vi "save_tracks_to_mat.vi"(3 "Max Spatial Drift Since Experiment Start (mm)":dbl, 5 "Max Spatial Drift Since Last Calibration (mm)":dbl, 7 "DecodedCameraFrames":i32[](array[numeric]), 8 "error in":errorcluster, 11 "Completed Tracks":T1[](array[typedef])) -> (0 "error out":errorcluster, 1 "Last Buffer":i32, 2 "total time elapsed (ms)":i32)   [LabVIEW 2019]
uses:
  WormTrackCluster.ctl
  StimulusObject.lvclass
  TrackTerminationReasonEnum.ctl
  WormTrackSavingCluster.ctl
  TimestampsFunctionalGlobalOperations.ctl
  <vilib>/addons/h5labview2/file/H5Fmode.ctl
  StimulusObject.lvclass/StimulusObject.ctl
  ParametersGlobal.vi
  <vilib>/addons/h5labview2/file/H5F.lvlib
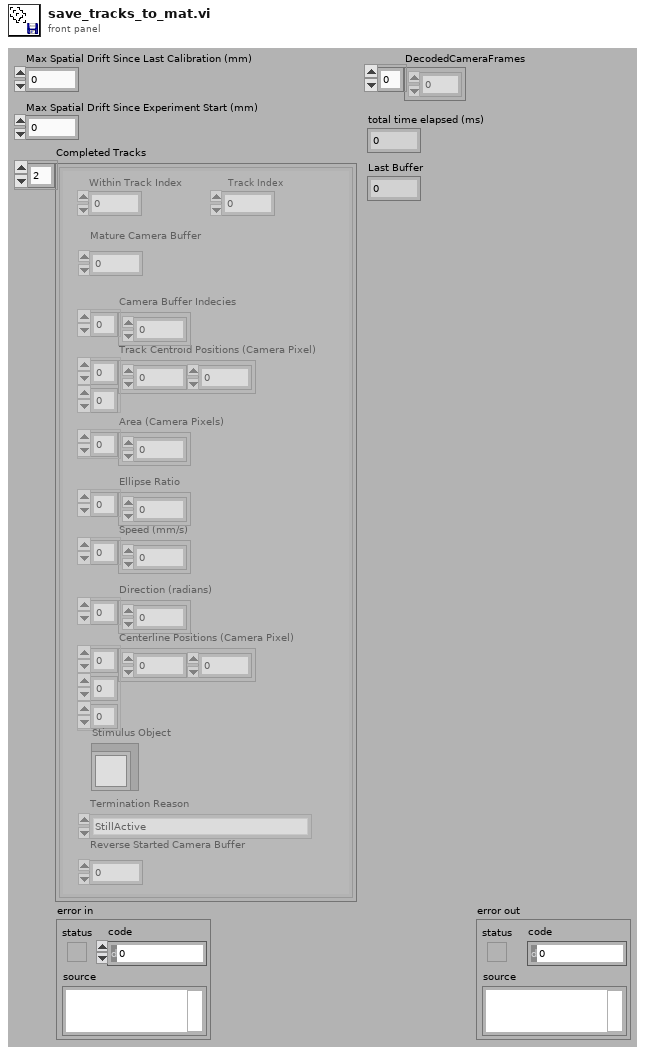
[diagram p1: front panel]
types:
  T1 = typedef "WormTrackCluster.ctl" = cluster{"Track Centroid Positions (Camera Pixel)":sgl[][], "Within Track Index":i32, "Camera Buffer Indecies":i32[], "Area (Camera Pixels)":i32[], "Speed (mm/s)":sgl[], "Direction (radians)":sgl[], "Centerline Positions (Camera Pixel)":sgl[][][], "Ellipse Ratio":sgl[], "Stimulus Object":refnum<class "StimulusObject.lvclass">, "Termination Reason":T2, "Track Index":i32, "Mature Camera Buffer":i32, "Reverse Started Camera Buffer":i32}
  T2 = typedef "TrackTerminationReasonEnum.ctl" = enum16{"StillActive", "MaxDisplacement", "NoBlobsLeft", "AreaIncrease", "AreaDecrease", "ExperimentEnded"}
  T3 = typedef "H5F.lvlib/H5Fmode.ctl" = enum16{"read-only", "read-write", "overwrite", "create new", "open or create"}
  T4 = typedef "TimestampsFunctionalGlobalOperations.ctl" = enum16{"Initialize", "Dump", "UpdateTime", "ReadTime"}
  T5 = typedef "WormTrackSavingCluster.ctl" = cluster{"Path":sgl[][], "Frames":i32[], "Size":i32[], "Speed":sgl[], "Direction":sgl[], "LabviewCenterline":sgl[][][], "EllipseRatio":sgl[], "TerminationReason":string, "WormIndex":i32, "MatureCameraBuffer":i32, "Stimulus":sgl[][]}
  T6 = typedef "IMAQ Image.ctl" = refnum<image>
  T7 = typedef "hid_t.ctl" = i32
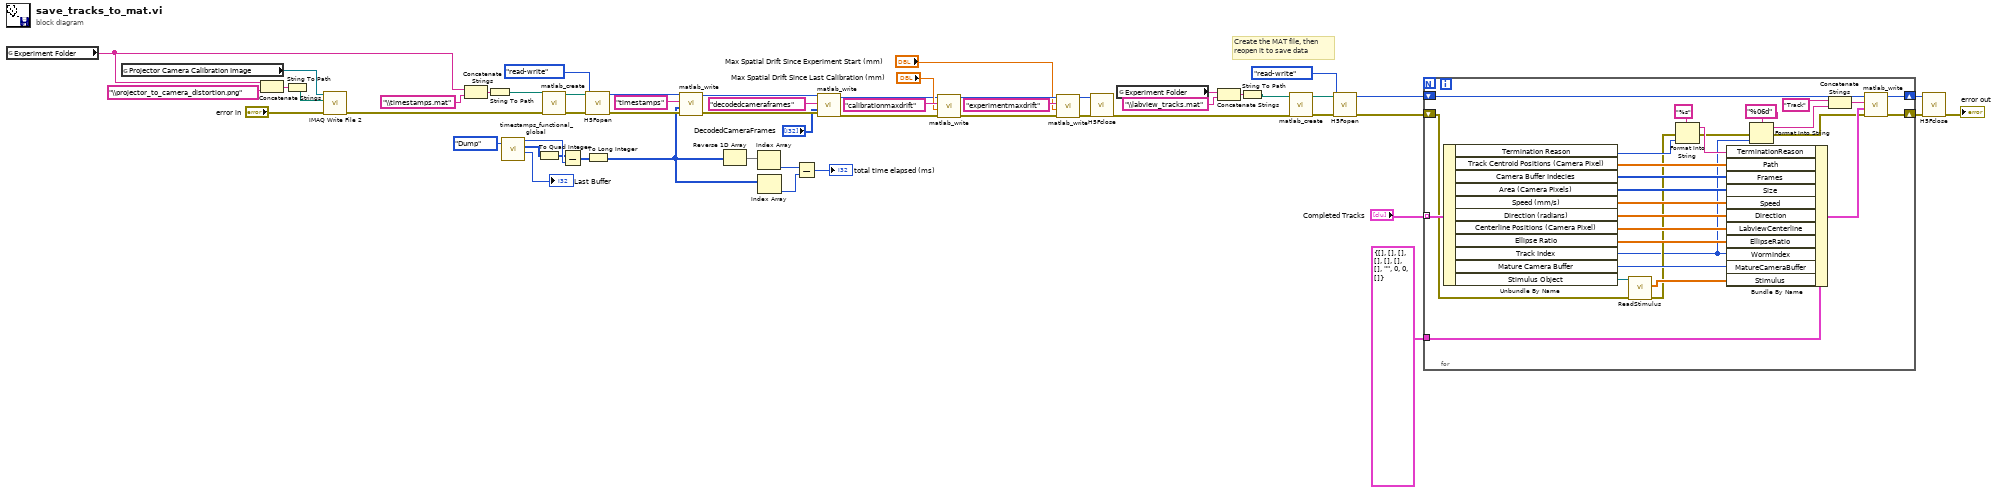
[diagram p0: block diagram]
diagram:
  # "Create the MAT file, then\nreopen it to save data"
  n1 = global read "ParametersGlobal.vi" "Experiment Folder"() -> (w11:string)
  n2 = global read "ParametersGlobal.vi" "Projector Camera Calibration Image"() -> (w13:T6)
  n3 = Concatenate Strings(w11, "\\projector_to_camera_distortion.png" ("string")) -> (w17:string)
  n4 = String To Path(string=w17) -> (path=w12:path)
  n5 = call-poly "IMAQ Write File 2"("error in (no error)"="error in", "File Path"=w12, "Image"=w13) -> ("error out"=w14:errorcluster)  [unwired: 7 in, 1 out]
  n6 = Concatenate Strings(w11, "\\timestamps.mat" ("string")) -> (w37:string)
  n7 = String To Path(string=w37) -> (path=w33:path)
  n8 = call "timestamps_functional_global.vi"("Operation"=TimestampsFunctionalGlobalOperations."Dump") -> ("Last Buffer"=→"Last Buffer":i32, "Timestamps"=w40:u32[], "Timestamp Out"=w41:u32)  [unwired: 4 in]
  n9 = To Quad Integer(1:w40) -> (0:w39:i64[])
  n10 = call "matlab_create.vi"("error in"=w14, "path in"=w33) -> ("error out"=w35:errorcluster, "path out"=w36:path)  [unwired: 4 in]
  n11 = Subtract(x=w39, y=w41) -> (x-y=w32:i64[])
  n12 = call <vilib>:"H5Fopen.vi"("error in (no error)"=w35, "mode (read-only)"=H5Fmode."read-write", "path"=w36) -> ("error out"=w29:errorcluster, "ref out"=w30:T7)  [unwired: 7 in]
  n13 = To Long Integer(number=w32) -> (32bit integer=w22:i32[])
  n14 = call "matlab_write.vi"("error in"=w29, "data in"=w22, "name"="timestamps", "ref in"=w30) -> ("error out"=w26:errorcluster, "ref out"=w25:T7)  [unwired: 2 in]
  n15 = Reverse 1D Array(array=w22) -> (reversed array=w23:i32[])
  n16 = Index Array(array=w23) -> (element=w21:i32)  [unwired: 1 in]
  n17 = Index Array(array=w22) -> (element=w20:i32)  [unwired: 1 in]
  n18 = Subtract(x=w21, y=w20) -> (x-y=→"total time elapsed (ms)":i32)
  n19 = call "matlab_write.vi"("error in"=w26, "data in"="DecodedCameraFrames", "name"="decodedcameraframes", "ref in"=w25) -> ("error out"=w8:errorcluster, "ref out"=w2:T7)  [unwired: 2 in]
  n20 = call "matlab_write.vi"("error in"=w8, "data in"="Max Spatial Drift Since Last Calibration (mm)", "name"="calibrationmaxdrift", "ref in"=w2) -> ("error out"=w6:errorcluster, "ref out"=w3:T7)  [unwired: 2 in]
  n21 = call "matlab_write.vi"("error in"=w6, "data in"="Max Spatial Drift Since Experiment Start (mm)", "name"="experimentmaxdrift", "ref in"=w3) -> ("error out"=w5:errorcluster, "ref out"=w4:T7)  [unwired: 2 in]
  n22 = call <vilib>:"H5Fclose.vi"("error in (no error)"=w5, "ref"=w4) -> ("error out"=w31:errorcluster)  [unwired: 9 in]
  n23 = global read "ParametersGlobal.vi" "Experiment Folder"() -> (w48:string)
  n24 = Concatenate Strings(w48, "\\labview_tracks.mat" ("string")) -> (w46:string)
  n25 = String To Path(string=w46) -> (path=w45:path)
  n26 = call "matlab_create.vi"("error in"=w31, "path in"=w45) -> ("error out"=w55:errorcluster, "path out"=w56:path)  [unwired: 4 in]
  n27 = call <vilib>:"H5Fopen.vi"("error in (no error)"=w55, "mode (read-only)"=H5Fmode."read-write", "path"=w56) -> ("error out"=w51:errorcluster, "ref out"=w52:T7)  [unwired: 7 in]
  n28 = for {
    shift-right: [w82] -> w49
    shift-left: w52 -> [w84]
    shift-right: [w83] -> w50
    shift-left: w51 -> [w63]
    tunnel: "Completed Tracks" -> [w79] mode=indexing
    tunnel: T5 {"Path"=[], "Frames"=[], "Size"=[], "Speed"=[], "Direction"=[], "LabviewCenterline"=[], "EllipseRatio"=[], "TerminationReason"="", "WormIndex"=0, "MatureCameraBuffer"=0, "Stimulus"=[]} ("Tracks") -> [w78]
    n29 = Unbundle By Name(w79) -> ("Termination Reason"=w68:T2, "Track Centroid Positions (Camera Pixel)"=w77:sgl[][], "Camera Buffer Indecies"=w76:i32[], "Area (Camera Pixels)"=w75:i32[], "Speed (mm/s)"=w74:sgl[], "Direction (radians)"=w73:sgl[], "Centerline Positions (Camera Pixel)"=w72:sgl[][][], "Ellipse Ratio"=w71:sgl[], "Track Index"=w58:i32, "Mature Camera Buffer"=w70:i32, "Stimulus Object"=w66:refnum<class "StimulusObject.lvclass">)
    n30 = call "ReadStimulus.vi"("error in (no error)"=w63, "StimulusObject in"=w66) -> ("error out"=w62:errorcluster, "StimulusOut"=w65:sgl[][])  [unwired: 7 in, 1 out]
    n31 = Format Into String(format string="%s", error in=w62, w68) -> (resulting string=w67:string, error out=w60:errorcluster)  [unwired: 1 in]
    n32 = Bundle By Name(cluster=w78, "TerminationReason"=w67, "Path"=w77, "Frames"=w76, "Size"=w75, "Speed"=w74, "Direction"=w73, "LabviewCenterline"=w72, "EllipseRatio"=w71, "WormIndex"=w58, "MatureCameraBuffer"=w70, "Stimulus"=w65) -> (w64:T5)
    n33 = Format Into String(format string="%06d" ("string"), error in=w60, w58) -> (resulting string=w57:string, error out=w59:errorcluster)  [unwired: 1 in]
    n34 = Concatenate Strings("Track" ("name"), w57) -> (w80:string)
    n35 = call "matlab_write.vi"("error in"=w59, "data in"=w64, "name"=w80, "ref in"=w84) -> ("error out"=w83:errorcluster, "ref out"=w82:T7)  [unwired: 2 in]
  }
  n36 = call <vilib>:"H5Fclose.vi"("error in (no error)"=w50, "ref"=w49) -> ("error out"=→"error out":errorcluster)  [unwired: 9 in]
